vi "DSSwithMyDAQ.vi"() -> ()   [LabVIEW 2023]
uses:
  Controls/Keys.ctl
  Controls/States.ctl
  Controls/DAQ Actions.ctl
panel:
  out "LEDs":u32[](array[colorbox])
  out "Present state":T1
  in  "STOP":bool
  out "Reset":bool
  out "Keys":T2 caption="Keys inputs"
  # "K1    K2"
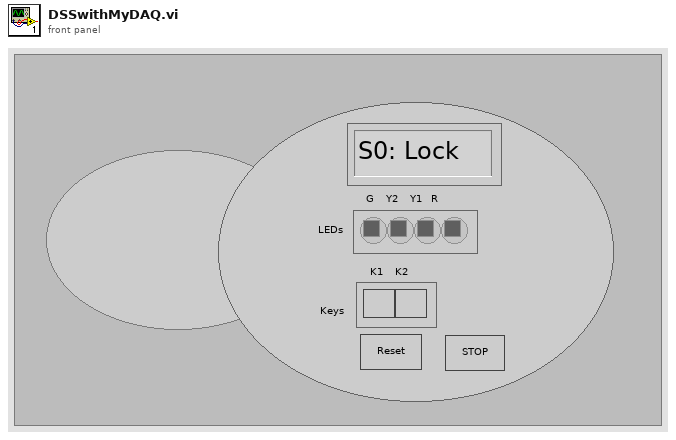
[diagram p1: front panel]
types:
  T1 = typedef "states.ctl" = enum16{"S0: Lock", "S1: Processing1 ", "S2: Processing2", "S3: Processing3", "S4: Unlock"}
  T2 = typedef "Keys.ctl" = bool[]
  T3 = typedef "DAQ Actions.ctl" = enum16{"Initialize DAQ", "Read Keys", "Read Reset ", "Write LEDs", "Release DAQ"}
  T4 = typedef "States.ctl" = enum16{"S0: Lock", "S1: Processing1 ", "S2: Processing2", "S3: Processing3", "S4: Unlock"}
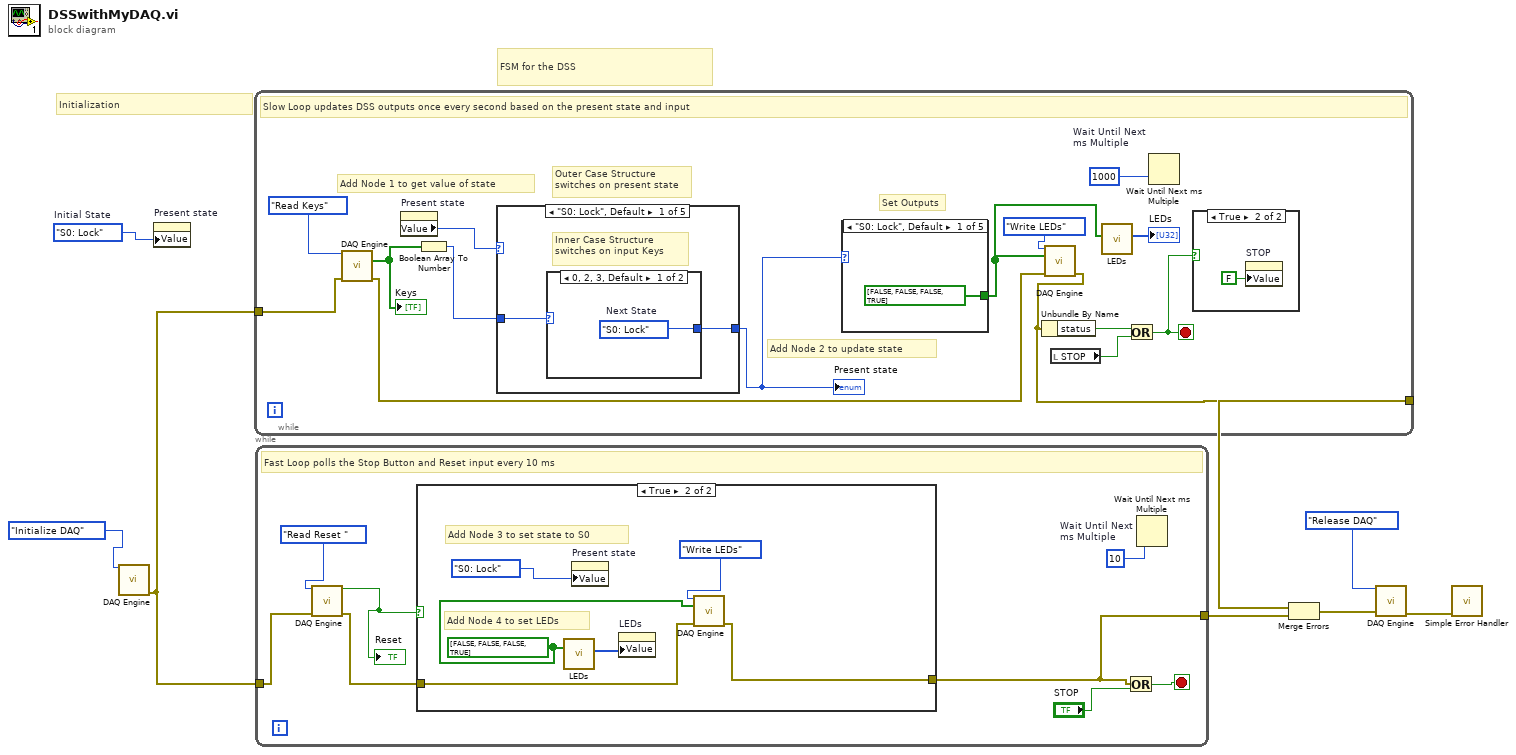
[diagram p0: block diagram]
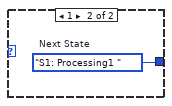
[diagram p4: hidden frame]
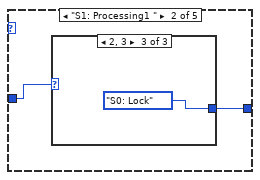
[diagram p5: hidden frame]
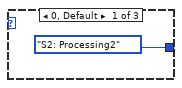
[diagram p6: hidden frame]
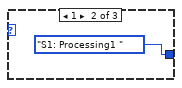
[diagram p7: hidden frame]
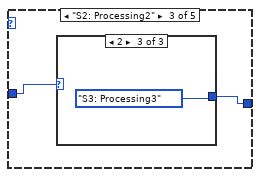
[diagram p8: hidden frame]
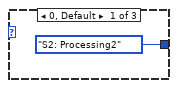
[diagram p9: hidden frame]
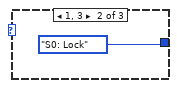
[diagram p10: hidden frame]
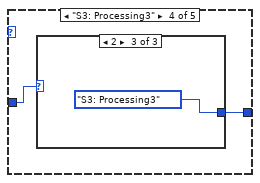
[diagram p11: hidden frame]
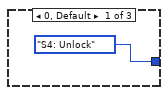
[diagram p12: hidden frame]
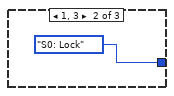
[diagram p13: hidden frame]
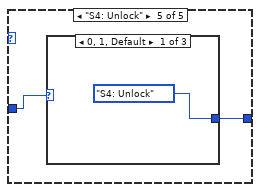
[diagram p14: hidden frame]
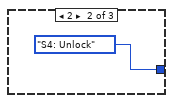
[diagram p15: hidden frame]
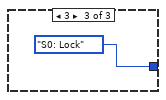
[diagram p16: hidden frame]
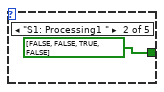
[diagram p17: hidden frame]
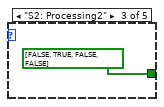
[diagram p18: hidden frame]
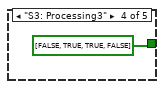
[diagram p19: hidden frame]
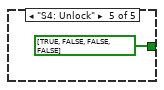
[diagram p20: hidden frame]
diagram:
  w8 = states."S0: Lock"  # Initial State
  # "Initialization"
  # "FSM for the DSS"
  n1 = call "DAQ Engine.vi"("DAQ Action"=DAQ_Actions."Initialize DAQ") -> ("Error Out"=w4:errorcluster)  [unwired: 12 in, 2 out]
  n2 = property on="Present state" class="Enum (strict)"("Value"=w8) -> ()  [unwired: 2 in, 2 out]
  n3 = while {
    tunnel: w4 -> [w14]
    tunnel: [w11] -> w6
    stop <- w17 stop-if-true
    # "Add Node 2 to update state"
    # "Add Node 1 to get value of state"
    # "Set Outputs"
    # "Outer Case Structure \nswitches on present state"
    # "Slow Loop updates DSS outputs once every second based on the present state and input"
    n4 = call "DAQ Engine.vi"("DAQ Action"=DAQ_Actions."Read Keys", "Error In"=w14) -> ("Keys"=w16:T2, "Error Out"=w12:errorcluster)  [unwired: 11 in, 1 out]
    "Keys" <- w16
    n5 = property on="Present state" class="Enum (strict)"() -> ("Value"=w18:T1)  [unwired: 2 in, 2 out]
    n6 = Boolean Array To Number(Boolean array=w16) -> (number=w20:u32)
    n7 = case shown="\"S0: Lock\", Default" w18 {
      tunnel: [w26 w29 w34 w39 w44] -> w19
      tunnel: w20 -> [w25 w30 w35 w40 w45]
      frame "S0: Lock", Default {
        # "Inner Case Structure \nswitches on input Keys"
        n8 = case shown="0, 2, 3, Default" w25 {
          tunnel: [w27 w28] -> w26
          frame 0, 2, 3, Default {
            w27 = states."S0: Lock"  # Next State
          }
          frame 1 {
            w28 = states."S1: Processing1 "  # Next State
          }
        }
      }
      frame "S1: Processing1 " {
        n9 = case shown="2, 3" w30 {
          tunnel: [States."S2: Processing2" ("State") States."S1: Processing1 " ("State") States."S0: Lock" ("State")] -> w29
          frame 0, Default {
          }
          frame 1 {
          }
          frame 2, 3 {
          }
        }
      }
      frame "S2: Processing2" {
        n10 = case shown="2" w35 {
          tunnel: [States."S2: Processing2" ("State") States."S0: Lock" ("State") States."S3: Processing3" ("State")] -> w34
          frame 0, Default {
          }
          frame 1, 3 {
          }
          frame 2 {
          }
        }
      }
      frame "S3: Processing3" {
        n11 = case shown="2" w40 {
          tunnel: [States."S4: Unlock" ("State") States."S0: Lock" ("State") States."S3: Processing3" ("State")] -> w39
          frame 0, Default {
          }
          frame 1, 3 {
          }
          frame 2 {
          }
        }
      }
      frame "S4: Unlock" {
        n12 = case shown="0, 1, Default" w45 {
          tunnel: [States."S4: Unlock" ("State") States."S4: Unlock" ("State") States."S0: Lock" ("State")] -> w44
          frame 0, 1, Default {
          }
          frame 2 {
          }
          frame 3 {
          }
        }
      }
    }
    "Present state" <- w19
    n13 = case shown="\"S0: Lock\", Default" w19 {
      tunnel: [bool[] [FALSE, FALSE, FALSE, TRUE] bool[] [FALSE, FALSE, TRUE, FALSE] ("LEDs") bool[] [FALSE, TRUE, FALSE, FALSE] ("LEDs") bool[] [FALSE, TRUE, TRUE, FALSE] ("LEDs") bool[] [TRUE, FALSE, FALSE, FALSE] ("LEDs")] -> w9
      frame "S0: Lock", Default {
      }
      frame "S1: Processing1 " {
      }
      frame "S2: Processing2" {
      }
      frame "S3: Processing3" {
      }
      frame "S4: Unlock" {
      }
    }
    n14 = call "DAQ Engine.vi"("DAQ Action"=DAQ_Actions."Write LEDs", "LEDs"=w9, "Error In"=w12) -> ("Error Out"=w11:errorcluster)  [unwired: 10 in, 2 out]
    n15 = Unbundle By Name "Unbundle By Name"(w11) -> ("status"=w22:bool)
    n16 = local read "STOP"() -> (w23:bool)
    n17 = call "LEDs.vi"("Array"=w9) -> ("Array 2"=→"LEDs":u32[])  [unwired: 10 in]
    n18 = Or(x=w22, y=w23) -> (x .or. y?=w17:bool)
    n19 = Wait Until Next ms Multiple "Wait Until Next \nms Multiple"(millisecond multiple=u32 1000) -> ()  [unwired: 1 out]
    n20 = case shown="True" w17 {
      frame False {
      }
      frame True {
        n21 = property on="STOP" class="Bool (strict)"("Value"=FALSE ("STOP")) -> ()  [unwired: 2 in, 2 out]
      }
    }
  }
  n22 = while {
    tunnel: w4 -> [w55]
    tunnel: [w59] -> w7
    stop <- w61 stop-if-true
    # "Fast Loop polls the Stop Button and Reset input every 10 ms"
    n23 = call "DAQ Engine.vi"("DAQ Action"=DAQ_Actions."Read Reset ", "Error In"=w55) -> ("Reset"=w56:bool, "Error Out"=w54:errorcluster)  [unwired: 11 in, 1 out]
    "Reset" <- w56
    n24 = case shown="True" w56 {
      tunnel: w54 -> [w62 w65]
      tunnel: [w62 w64] -> w59
      frame False {
      }
      frame True {
        w63 = bool[] [FALSE, FALSE, FALSE, TRUE]
        # "Add Node 4 to set LEDs"
        # "Add Node 3 to set state to S0"
        n25 = call "LEDs.vi"("Array"=w63) -> ("Array 2"=w67:u32[])  [unwired: 10 in]
        n26 = property on="Present state" class="Enum (strict)"("Value"=States."S0: Lock" ("State")) -> ()  [unwired: 2 in, 2 out]
        n27 = property on="LEDs" class="Arr (strict)"("Value"=w67) -> ()  [unwired: 2 in, 2 out]
        n28 = call "DAQ Engine.vi"("DAQ Action"=DAQ_Actions."Write LEDs", "LEDs"=w63, "Error In"=w65) -> ("Error Out"=w64:errorcluster)  [unwired: 10 in, 2 out]
      }
    }
    n29 = Or(x=w59, y="STOP") -> (x .or. y?=w61:bool)
    n30 = Wait Until Next ms Multiple "Wait Until Next \nms Multiple"(millisecond multiple=u32 10) -> ()  [unwired: 1 out]
  }
  n31 = Merge Errors(w6, w7) -> (w2:errorcluster)
  n32 = call "DAQ Engine.vi"("DAQ Action"=DAQ_Actions."Release DAQ", "Error In"=w2) -> ("Error Out"=w1:errorcluster)  [unwired: 11 in, 2 out]
  n33 = call <vilib>:"Simple Error Handler.vi"("error in (no error)"=w1) -> ()  [unwired: 4 in, 5 out]
